vi "Wiimote Parse IR Sensor.vi"(8 "error in":errorcluster, 11 "pReportBuffer in":u8[](array[numeric]) format="%02x") -> (0 "error out":errorcluster, 3 "Wiimote IR Sensor out":T1)   [LabVIEW 2011, in "Wiimote.lvlib"]
uses:
  Wiimote.lvlib
  Wiimote IR Sensor.ctl
  Wiimote Point.ctl
panel:
  in  "Wiimote IR Sensor":T1
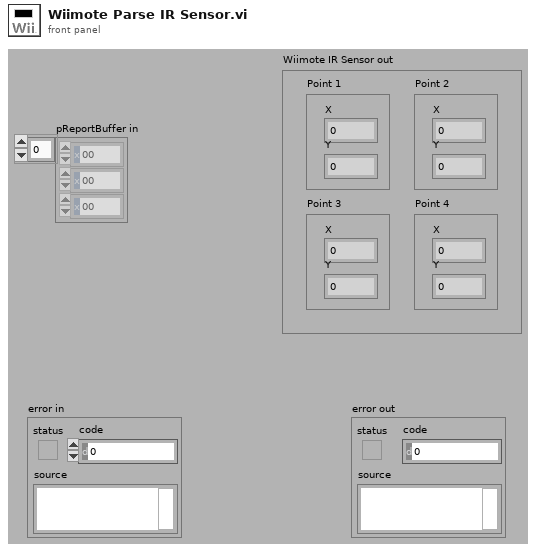
[diagram p1: front panel]
types:
  T1 = typedef "Wiimote.lvlib/Wiimote IR Sensor.ctl" = cluster{"Point 1":T2, "Point 2":T2, "Point 3":T2, "Point 4":T2}
  T2 = typedef "Wiimote.lvlib/Wiimote Point.ctl" = cluster{"X":u16, "Y":u16}
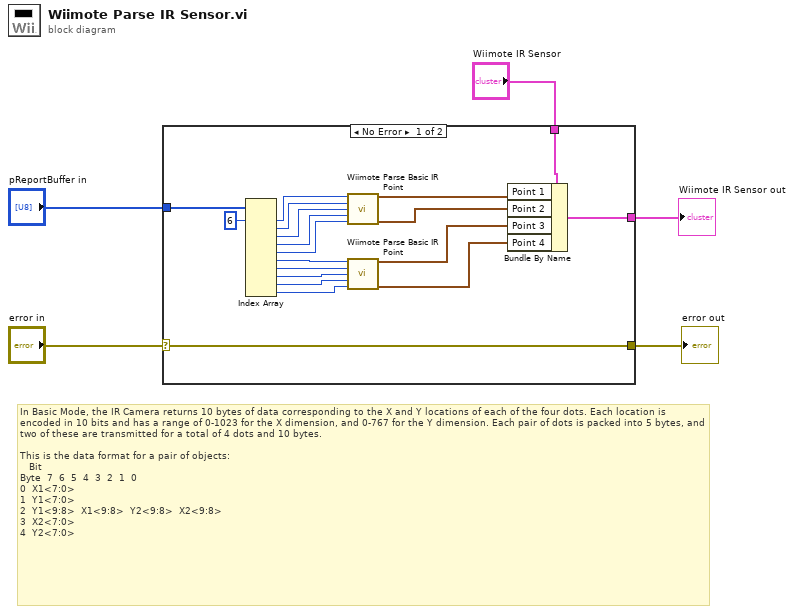
[diagram p0: block diagram]
diagram:
  # "In Basic Mode, the IR Camera returns 10 bytes of data corresponding to the X and Y locations of each of the four dots. Each location is encoded in 10 bits and has a range of 0-1023 for the X dimension, and 0-767 for the Y dimension. Each pair of dots is packed into 5 bytes, and two of these are transmitted for a total of 4 dots and 10 bytes.\n\nThis is the data format for a pair of objects:\n  \tBit\nByte \t7 \t6 \t5 \t4 \t3 \t2 \t1 \t0\n0 \tX1<7:0>\n1 \tY1<7:0>\n2 \tY1<9:8> \tX1<9:8> \tY2<9:8> \tX2<9:8>\n3 \tX2<7:0>\n4 \tY2<7:0>"
  n1 = case shown="No Error" "error in" {
    selector: "error in" -> [w24 w25]
    tunnel: [w24 w25] -> w4
    tunnel: "pReportBuffer in" -> [w23 _]
    tunnel: "Wiimote IR Sensor" -> [w21 _]
    tunnel: [w20 _] -> w1
    frame No Error {
      n2 = Index Array(array=w23, index #1=6 ("index")) -> (element #1=w17:u8, element #2=w16:u8, element #3=w15:u8, element #4=w14:u8, element #5=w13:u8, element #6=w12:u8, element #7=w11:u8, element #8=w10:u8, element #9=w9:u8, element #10=w8:u8)  [unwired: 9 in]
      n3 = call "Wiimote Parse Basic IR Point.vi"("Byte 0 in"=w17, "Byte 1 in"=w16, "Byte 2 in"=w15, "Byte 3 in"=w14, "Byte 4 in"=w13) -> ("Wiimote Point 1 out"=w19:T2, "Wiimote Point 2 out"=w18:T2)  [unwired: 9 in]
      n4 = call "Wiimote Parse Basic IR Point.vi"("Byte 0 in"=w12, "Byte 1 in"=w11, "Byte 2 in"=w10, "Byte 3 in"=w9, "Byte 4 in"=w8) -> ("Wiimote Point 1 out"=w7:T2, "Wiimote Point 2 out"=w6:T2)  [unwired: 9 in]
      n5 = Bundle By Name(cluster=w21, "Point 1"=w19, "Point 2"=w18, "Point 3"=w7, "Point 4"=w6) -> (w20:T1)
    }
    frame Error {
    }
  }
  "error out" <- w4
  "Wiimote IR Sensor out" <- w1
